vi "Create.vi"(8 "error in (no error)":errorcluster, 10 "Group Buffer":refnum<class "Group Buffer DBL.lvclass">) -> (0 "error out":errorcluster, 3 "Group Data Handler out":refnum<class "Group Data Handler.lvclass">)   [LabVIEW 2020, in "VolatusHistorian.lvlib" / "Group Data Handler.lvclass"]
uses:
  Group Data Handler.lvclass
  Group Buffer DBL/Group Buffer DBL.lvclass
  Group Data Handler.lvclass/Group Data Handler.ctl
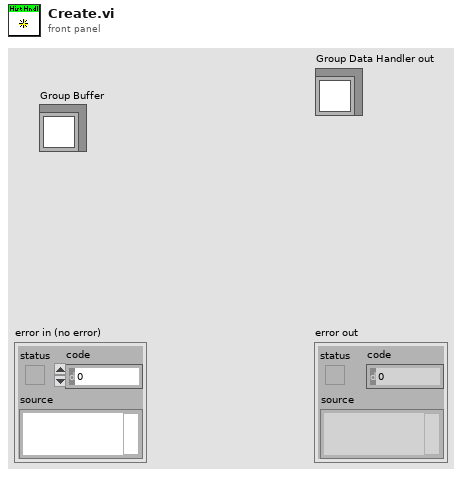
[diagram p1: front panel]
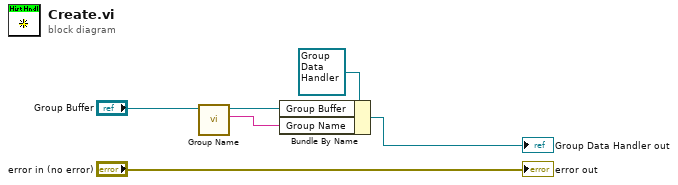
[diagram p0: block diagram]
diagram:
  n1 = call "Group Name.vi"("Group Buffer DBL in"="Group Buffer") -> ("Name"=w1:string, "Group Buffer DBL out"=w2:refnum<class "Group Buffer DBL.lvclass">)  [unwired: 8 in, 1 out]
  n2 = Bundle By Name(cluster=refnum<class "Group Data Handler.lvclass"> refnum ("Group Data Handler in"), "Group Buffer"=w2, "Group Name"=w1) -> (→"Group Data Handler out":refnum<class "Group Data Handler.lvclass">)
  "error out" <- "error in (no error)"
